vi "String.Append Item to String List.vi"(5 "Delimiter":string=", ", 7 "Prefix":string="Missing: ", 10 "New Data":string, 11 "Existing Str":string) -> (3 "New Str":string)   [LabVIEW 2018]
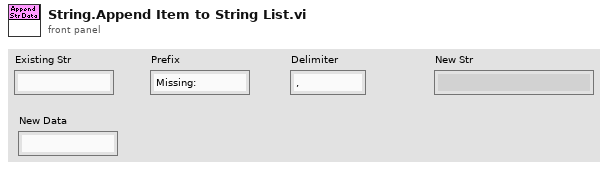
[diagram p1: front panel]
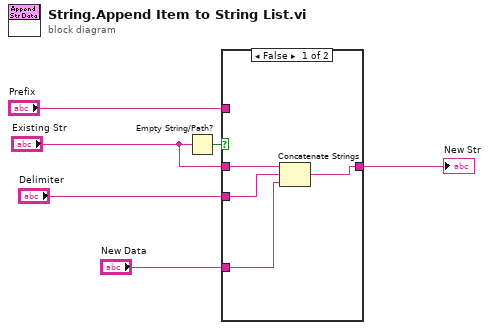
[diagram p0: block diagram]
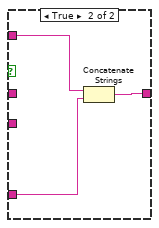
[diagram p2: hidden frame]
diagram:
  n1 = Empty String/Path?(string/path="Existing Str") -> (empty?=w6:bool)
  n2 = case shown="False" w6 {
    tunnel: "Existing Str" -> [w10 _]
    tunnel: [w8 w12] -> w3
    tunnel: "New Data" -> [w9 w13]
    tunnel: "Prefix" -> [_ w11]
    tunnel: "Delimiter" -> [w7 _]
    frame False {
      n3 = Concatenate Strings(w10, w7, w9) -> (w8:string)
    }
    frame True {
      n4 = Concatenate Strings(w11, w13) -> (w12:string)
    }
  }
  "New Str" <- w3
